vi "Step-3-save-to-hp_state-i.vi"(8 "hp_state_in (u64)":u64[](array[numeric]) format="%.0x", 10 "j":u64, 11 "New-Val":u64[](array[numeric]) format="%.0x") -> (2 "hp_state_out (u64)":u64[](array[numeric]) format="%.0x")   [LabVIEW 2017]
panel:
  out "j/8":u64
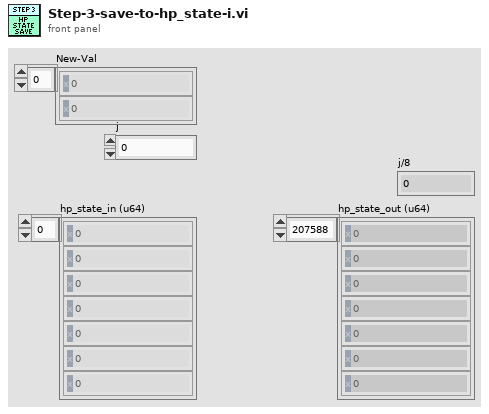
[diagram p1: front panel]
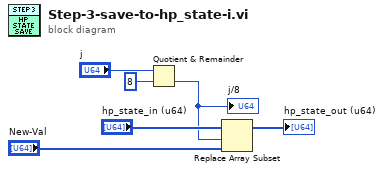
[diagram p0: block diagram]
diagram:
  n1 = Quotient & Remainder(x="j", y=u64 8) -> (floor(x/y)=w3:u64)  [unwired: 1 out]
  "j/8" <- w3
  n2 = Replace Array Subset(array="hp_state_in (u64)", new element="New-Val", index=w3) -> (→"hp_state_out (u64)":u64[])
